vi "Query Multi Eval Meas List ACLR UTRA Limit Check Results.vi"(6 "UTRA Channel (First adjacent)":T1=1 items=["First adjacent"=1, "Second adjacent"=2], 7 "Carrier Frequency (Positive)":i32(ring)=1 items=["Negative", "Positive"], 8 "error in (no error)":errorcluster, 9 "Result Type (Current)":i32(ring) items=["Current", "Average"], 10 "Instance (1)":T2=1, 11 "VISA resource name":refnum<visa-resource-name>) -> (0 "error out":errorcluster, 1 "Limit Check Results":i32[](array[numeric]), 2 "Reliability":i32, 3 "VISA resource name out":refnum<visa-resource-name>)   [LabVIEW 2020, in "Rohde&Schwarz CMWXP NR FR1 Measurement.lvlib"]
doc: "Return the ACLR limit check results for the first or second adjacent UTRA channel above (Positive) or below (Negative) the carrier frequency for all measured list mode segments.\n\nAttributes:\nRSCMWXPNRFR1M_ATTR_QUERY_MULTI_EVAL_MEAS_LIST_ACLR_UTRA_NEGATIVE_CURRENT_LIMIT_CHECK_RESULTS\nRSCMWXPNRFR1M_ATTR_QUERY_MULTI_EVAL_MEAS_LIST_ACLR_UTRA_NEGATIVE_AVERAGE_LIMIT_CHECK_RESULTS\nRSCMWXPNRFR1M_ATTR_QUERY_MULTI_EVAL_MEAS_LIST_ACLR_UTRA_POSITIVE_CURRENT_LIMIT_CHECK_RESULTS\nRSCMWXPNRFR1M_ATTR_QUERY_MULTI_EVAL_MEAS_LIST_ACLR_UTRA_POSITIVE_AVERAGE_LIMIT_CHECK_RESULTS\n\nRemote-control commands:\nCALCulate:NRSub:MEAS<i>:MEValuation:LIST:ACLR:UTRA<no>:NEGativ:CURRent?\nCALCulate:NRSub:MEAS<i>:MEValuation:LIST:ACLR:UTRA<no>:NEGativ:AVERage?\nCALCulate:NRSub:MEAS<i>:MEValuation:LIST:ACLR:UTRA<no>:POSitiv:CURRent?\nCALCulate:NRSub:MEAS<i>:MEValuation:LIST:ACLR:UTRA<no>:POSitiv:AVERage?"
uses:
  <instrlib>/Rohde&Schwarz CMWXP NR FR1 Measurement/Rohde&Schwarz CMWXP NR FR1 Measurement.lvlib
  <instrlib>/Rohde&Schwarz CMWXP NR FR1 Measurement/Private/_Instance.ctl
  <instrlib>/Rohde&Schwarz CMWXP NR FR1 Measurement/Private/_UTRA.ctl
  <instrlib>/Rohde&Schwarz CMWXP NR FR1 Measurement/Private/rsidr_core.llb/rsidr_core.lvlib
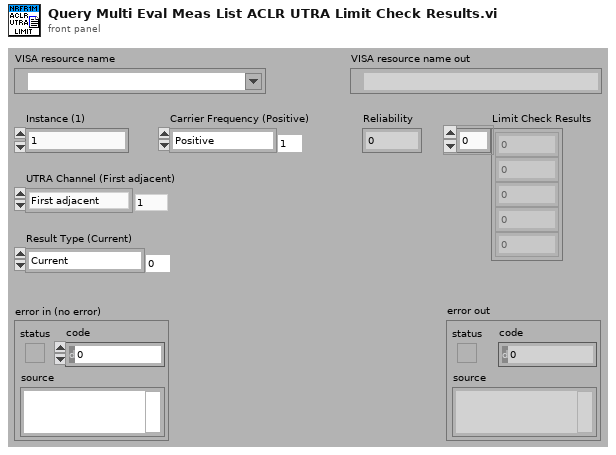
[diagram p1: front panel]
types:
  T1 = typedef "Rohde&Schwarz CMWXP NR FR1 Measurement.lvlib/_UTRA.ctl" = i32
  T2 = typedef "Rohde&Schwarz CMWXP NR FR1 Measurement.lvlib/_Instance.ctl" = i32
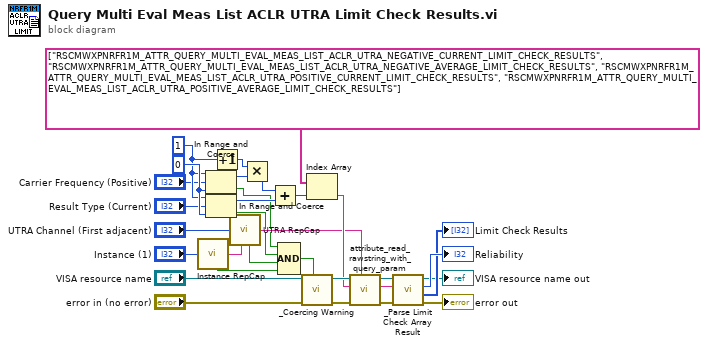
[diagram p0: block diagram]
diagram:
  w15 = 1
  w17 = 0
  n1 = call <instrlib>:"Instance RepCap.vi"("Instance In"="Instance (1)") -> ("In Range?"=w22:bool, "RepCap Identifier Out"=w21:string)  [unwired: 1 in]
  n2 = In Range and Coerce(upper limit=w15, x="Carrier Frequency (Positive)", lower limit=w17) -> (coerced(x)=w16:i32, In Range?=w11:bool)
  n3 = In Range and Coerce(upper limit=w15, x="Result Type (Current)", lower limit=w17) -> (coerced(x)=w18:i32, In Range?=w12:bool)
  n4 = Increment(x=w15) -> (x+1=w14:i32)
  n5 = call <instrlib>:"UTRA RepCap.vi"("UTRA In"="UTRA Channel (First adjacent)", "RepCap String In (\"\")"=w21) -> ("In Range?"=w20:bool, "RepCap Identifier Out"=w19:string)
  n6 = Multiply(x=w14, y=w16) -> (x*y=w13:i32)
  n7 = Add(x=w13, y=w18) -> (x+y=w30:i32)
  n8 = Compound Arithmetic op=AND(w11, w12, w20, w22) -> (w23:bool)
  n9 = call <instrlib>:"_Coercing Warning.vi"("In Range?"=w23, "error in (no error)"="error in (no error)", "VISA resource name"="VISA resource name") -> ("error out"=w27:errorcluster, "VISA resource name out"=w29:refnum<visa-resource-name>)  [unwired: 7 in]
  n10 = Index Array(array=string[] ["RSCMWXPNRFR1M_ATTR_QUERY_MULTI_EVAL_MEAS_LIST_ACLR_UTRA_NEGATIVE_CURRENT_LIMIT_CHECK_RESULTS", "RSCMWXPNRFR1M_ATTR_QUERY_MULTI_EVAL_MEAS_LIST_ACLR_UTRA_NEGATIVE_AVERAGE_LIMIT_CHECK_RESULTS", "RSCMWXPNRFR1M_ATTR_QUERY_MULTI_EVAL_MEAS_LIST_ACLR_UTRA_POSITIVE_CURRENT_LIMIT_CHECK_RESULTS", "RSCMWXPNRFR1M_ATTR_QUERY_MULTI_EVAL_MEAS_LIST_ACLR_UTRA_POSITIVE_AVERAGE_LIMIT_CHECK_RESULTS"], index=w30) -> (element=w28:string)
  n11 = call <instrlib>:"attribute_read_rawstring_with_query_param.vi"("Repeated Capability"=w19, "error in"=w27, "Attribute ID"=w28, "VISA resource name"=w29) -> ("error out"=w26:errorcluster, "Raw String out"=w25:string, "VISA resource name out"=w24:refnum<visa-resource-name>)  [unwired: 5 in]
  n12 = call <instrlib>:"_Parse Limit Check Array Result.vi"("error in (no error)"=w26, "Input String"=w25, "VISA resource name"=w24) -> ("error out"=→"error out":errorcluster, "Results"=→"Limit Check Results":i32[], "Reliability"=→"Reliability":i32, "VISA resource name out"=→"VISA resource name out":refnum<visa-resource-name>)  [unwired: 3 in, 1 out]
